vi "Comments and Commas.vi"() -> ()   [LabVIEW 2019]
doc: "An example of support for Comments and \"sloppy\" commas.\n\nThis is meant for hand-editted JSON files, where comments are useful, and there are mistakes made in placing commas.\n\n// Supports Comments\n{\n \"a\":1 // like this\n \"b\":2 /*or this style\n of multiline comment*/\n \"c\": 3 //oh, and notice I'm forgetting some commas\n \"d\":4, // except I've left a trailing one at the end\n}"
uses:
  d76af1bc-a9a6-4339-800b-d04741a931ff.vi
  vi.lib/JDP Science/JSONtext/Find Multiple Items.vi
  vi.lib/JDP Science/JSONtext/String Subset.vi
  vi.lib/JDP Science/JSONtext/support/Strip Quotes and Unescape.vi
  vi.lib/JDP Science/JSONtext/support/Unescape JSON string.vi
  vi.lib/JDP Science/JSONtext/Parsing/Parse Full Path or Item Name.vi
  vi.lib/JDP Science/JSONtext/Offset/Find Item Locations by Path.vi
  vi.lib/JDP Science/JSONtext/JSON text to Variant.vi
  vi.lib/JDP Science/JSONtext/LVClass Serializer/JSONtext LVClass Serializer.lvclass
  vi.lib/JDP Science/JSONtext/JSONtext.lvlib
panel:
  out "<JSON>":string
  out "All functions should work, ignoring comments":i32[](array[numeric])
  in  "JSON with comments and sloppy commas":string="// Supports Comments\n{\n    \"a\":1    // like this\n    \"b\":2   /*or this style\n                 of multiline comment*/\n    \"c\": 3  //oh, and notice I'm forgetting some commas\n    \"d\":4, // except I've left a trailing one at the end\n}"
  out "<JSON>Reformat strips comments and fixes commas":string
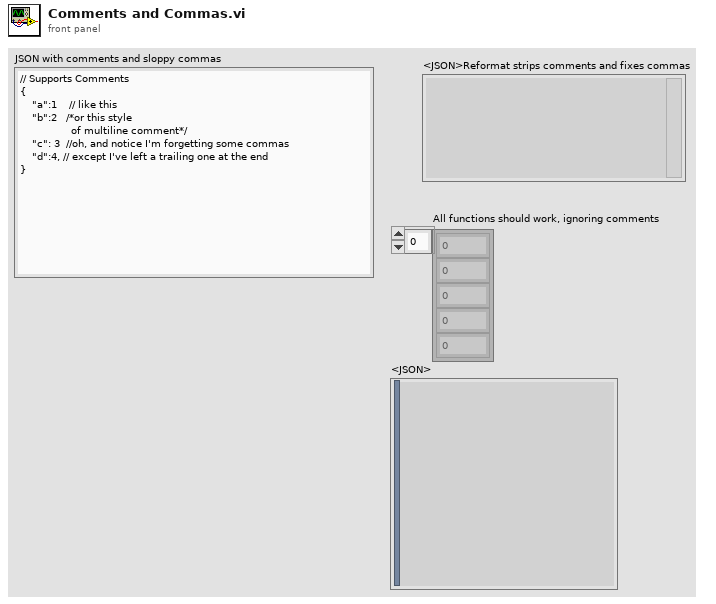
[diagram p1: front panel]
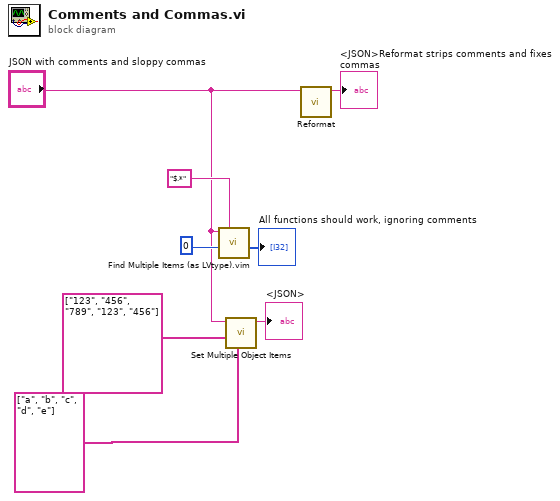
[diagram p0: block diagram]
diagram:
  n1 = call "Find Multiple Items (as LVtype).vim"("$Path or Item Name"="$.*", "Data Type and Default Value"=0, "JSON"="JSON with comments and sloppy commas") -> ("Array of Data"=→"All functions should work, ignoring comments":i32[])  [unwired: 5 in, 3 out]
  n2 = call "Set Multiple Object Items.vi"("Item Names"=string[] ["a", "b", "c", "d", "e"], "JSON Items"=string[] ["123", "456", "789", "123", "456"] ("Item Names"), "JSON"="JSON with comments and sloppy commas") -> ("<JSON>"=→"<JSON>":string)  [unwired: 6 in, 1 out]
  n3 = call "Reformat.vi"("JSON"="JSON with comments and sloppy commas") -> ("<JSON>"=→"<JSON>Reformat strips comments and fixes commas":string)  [unwired: 7 in, 3 out]
